vi "Pade_filter_parameters.vi"(7 "Cheby constraints":bool=TRUE, 10 "order cluster":cluster{u32, i32, i32}[][][](array[cluster])=[[[{3, 2, 2}, {3, 2, 1}, {0, 0, 0}, {0, 0, 0}, {0, 0, 0}, {0, 0, 0}, {0, 0, 0}], [{3, 3, 3}, {3, 3, 2}, {3, 3, 1}, {0, 0, 0}, {0, 0, 0}, {0, 0, 0}, {0, 0, 0}], [{3, 4, 4}, {3, 4, 3}, {3, 4, 2}, {3, 4, 1}, {0, 0, 0}, {0, 0, 0}, {0, 0, 0}], [{3, 5, 5}, {3, 5, 4}, {3, 5, 3}, {3, 5, 2}, {3, 5, 1}, {0, 0, 0}, {0, 0, 0}], [{3, 6, 6}, {3, 6, 5}, {3, 6, 4}, {3, 6, 3}, {3, 6, 2}, {3, 6, 1}, {0, 0, 0}], [{3, 7, 7}, {3, 7, 6}, {3, 7, 5}, {3, 7, 4}, {3, 7, 3}, {3, 7, 2}, {3, 7, 1}]], [[{4, 2, 2}, {4, 2, 1}, {0, 0, 0}, {0, 0, 0}, {0, 0, 0}, {0, 0, 0}, {0, 0, 0}], [{4, 3, 3}, {4, 3, 2}, {4, 3, 1}, {0, 0, 0}, {0, 0, 0}, {0, 0, 0}, {0, 0, 0}], [{4, 4, 4}, {4, 4, 3}, {4, 4, 2}, {4, 4, 1}, {0, 0, 0}, {0, 0, 0}, {0, 0, 0}], [{4, 5, 5}, {4, 5, 4}, {4, 5, 3}, {4, 5, 2}, {4, 5, 1}, {0, 0, 0}, {0, 0, 0}], [{4, 6, 6}, {4, 6, 5}, {4, 6, 4}, {4, 6, 3}, {4, 6, 2}, {4, 6, 1}, {0, 0, 0}], [{4, 7, 7}, {4, 7, 6}, {4, 7, 5}, {4, 7, 4}, {4, 7, 3}, {4, 7, 2}, {4, 7, 1}]], [[{5, 2, 2}, {5, 2, 1}, {0, 0, 0}, {0, 0, 0}, {0, 0, 0}, {0, 0, 0}, {0, 0, 0}], [{5, 3, 3}, {5, 3, 2}, {5, 3, 1}, {0, 0, 0}, {0, 0, 0}, {0, 0, 0}, {0, 0, 0}], [{5, 4, 4}, {5, 4, 3}, {5, 4, 2}, {5, 4, 1}, {0, 0, 0}, {0, 0, 0}, {0, 0, 0}], [{5, 5, 5}, {5, 5, 4}, {5, 5, 3}, {5, 5, 2}, {5, 5, 1}, {0, 0, 0}, {0, 0, 0}], [{5, 6, 6}, {5, 6, 5}, {5, 6, 4}, {5, 6, 3}, {5, 6, 2}, {5, 6, 1}, {0, 0, 0}], [{5, 7, 7}, {5, 7, 6}, {5, 7, 5}, {5, 7, 4}, {5, 7, 3}, {5, 7, 2}, {5, 7, 1}]], [[{6, 2, 2}, {6, 2, 1}, {0, 0, 0}, {0, 0, 0}, {0, 0, 0}, {0, 0, 0}, {0, 0, 0}], [{6, 3, 3}, {6, 3, 2}, {6, 3, 1}, {0, 0, 0}, {0, 0, 0}, {0, 0, 0}, {0, 0, 0}], [{6, 4, 4}, {6, 4, 3}, {6, 4, 2}, {6, 4, 1}, {0, 0, 0}, {0, 0, 0}, {0, 0, 0}], [{6, 5, 5}, {6, 5, 4}, {6, 5, 3}, {6, 5, 2}, {6, 5, 1}, {0, 0, 0}, {0, 0, 0}], [{6, 6, 6}, {6, 6, 5}, {6, 6, 4}, {6, 6, 3}, {6, 6, 2}, {6, 6, 1}, {0, 0, 0}], [{6, 7, 7}, {6, 7, 6}, {6, 7, 5}, {6, 7, 4}, {6, 7, 3}, {6, 7, 2}, {6, 7, 1}]], [[{7, 2, 2}, {7, 2, 1}, {0, 0, 0}, {0, 0, 0}, {0, 0, 0}, {0, 0, 0}, {0, 0, 0}], [{7, 3, 3}, {7, 3, 2}, {7, 3, 1}, {0, 0, 0}, {0, 0, 0}, {0, 0, 0}, {0, 0, 0}], [{7, 4, 4}, {7, 4, 3}, {7, 4, 2}, {7, 4, 1}, {0, 0, 0}, {0, 0, 0}, {0, 0, 0}], [{7, 5, 5}, {7, 5, 4}, {7, 5, 3}, {7, 5, 2}, {7, 5, 1}, {0, 0, 0}, {0, 0, 0}], [{7, 6, 6}, {7, 6, 5}, {7, 6, 4}, {7, 6, 3}, {7, 6, 2}, {7, 6, 1}, {0, 0, 0}], [{7, 7, 7}, {7, 7, 6}, {7, 7, 5}, {7, 7, 4}, {7, 7, 3}, {7, 7, 2}, {7, 7, 1}]], [[{8, 2, 2}, {8, 2, 1}, {0, 0, 0}, {0, 0, 0}, {0, 0, 0}, {0, 0, 0}, {0, 0, 0}], [{8, 3, 3}, {8, 3, 2}, {8, 3, 1}, {0, 0, 0}, {0, 0, 0}, {0, 0, 0}, {0, 0, 0}], [{8, 4, 4}, {8, 4, 3}, {8, 4, 2}, {8, 4, 1}, {0, 0, 0}, {0, 0, 0}, {0, 0, 0}], [{8, 5, 5}, {8, 5, 4}, {8, 5, 3}, {8, 5, 2}, {8, 5, 1}, {0, 0, 0}, {0, 0, 0}], [{8, 6, 6}, {8, 6, 5}, {8, 6, 4}, {8, 6, 3}, {8, 6, 2}, {8, 6, 1}, {0, 0, 0}], [{8, 7, 7}, {8, 7, 6}, {8, 7, 5}, {8, 7, 4}, {8, 7, 3}, {8, 7, 2}, {8, 7, 1}]], [[{9, 2, 2}, {9, 2, 1}, {0, 0, 0}, {0, 0, 0}, {0, 0, 0}, {0, 0, 0}, {0, 0, 0}], [{9, 3, 3}, {9, 3, 2}, {9, 3, 1}, {0, 0, 0}, {0, 0, 0}, {0, 0, 0}, {0, 0, 0}], [{9, 4, 4}, {9, 4, 3}, {9, 4, 2}, {9, 4, 1}, {0, 0, 0}, {0, 0, 0}, {0, 0, 0}], [{9, 5, 5}, {9, 5, 4}, {9, 5, 3}, {9, 5, 2}, {9, 5, 1}, {0, 0, 0}, {0, 0, 0}], [{9, 6, 6}, {9, 6, 5}, {9, 6, 4}, {9, 6, 3}, {9, 6, 2}, {9, 6, 1}, {0, 0, 0}], [{9, 7, 7}, {9, 7, 6}, {9, 7, 5}, {9, 7, 4}, {9, 7, 3}, {9, 7, 2}, {9, 7, 1}]], [[{10, 2, 2}, {10, 2, 1}, {0, 0, 0}, {0, 0, 0}, {0, 0, 0}, {0, 0, 0}, {0, 0, 0}], [{10, 3, 3}, {10, 3, 2}, {10, 3, 1}, {0, 0, 0}, {0, 0, 0}, {0, 0, 0}, {0, 0, 0}], [{10, 4, 4}, {10, 4, 3}, {10, 4, 2}, {10, 4, 1}, {0, 0, 0}, {0, 0, 0}, {0, 0, 0}], [{10, 5, 5}, {10, 5, 4}, {10, 5, 3}, {10, 5, 2}, {10, 5, 1}, {0, 0, 0}, {0, 0, 0}], [{10, 6, 6}, {10, 6, 5}, {10, 6, 4}, {10, 6, 3}, {10, 6, 2}, {10, 6, 1}, {0, 0, 0}], [{10, 7, 7}, {10, 7, 6}, {10, 7, 5}, {10, 7, 4}, {10, 7, 3}, {10, 7, 2}, {10, 7, 1}]], [[{11, 2, 2}, {11, 2, 1}, {0, 0, 0}, {0, 0, 0}, {0, 0, 0}, {0, 0, 0}, {0, 0, 0}], [{11, 3, 3}, {11, 3, 2}, {11, 3, 1}, {0, 0, 0}, {0, 0, 0}, {0, 0, 0}, {0, 0, 0}], [{11, 4, 4}, {11, 4, 3}, {11, 4, 2}, {11, 4, 1}, {0, 0, 0}, {0, 0, 0}, {0, 0, 0}], [{11, 5, 5}, {11, 5, 4}, {11, 5, 3}, {11, 5, 2}, {11, 5, 1}, {0, 0, 0}, {0, 0, 0}], [{11, 6, 6}, {11, 6, 5}, {11, 6, 4}, {11, 6, 3}, {11, 6, 2}, {11, 6, 1}, {0, 0, 0}], [{11, 7, 7}, {11, 7, 6}, {11, 7, 5}, {11, 7, 4}, {11, 7, 3}, {11, 7, 2}, {11, 7, 1}]]], 11 "Array":dbl[][][](array[numeric])=[[[0.002353454560863419, 0.007689391633254067, 99.0, 99.0, 99.0, 99.0, 99.0], [0.0023534545608634183, 0.0023534545608634183, nan, 99.0, 99.0, 99.0, 99.0], [0.002353454560863419, 0.0023534545608634187, 0.0023534545608634165, nan, 99.0, 99.0, 99.0], [0.0023534545608634187, 0.0023534545608634126, 0.0023534545608634187, nan, nan, 99.0, 99.0], [0.002353454560863415, 0.0023534545608634196, 0.0023534545608634187, 0.0023534545608634187, nan, nan, 99.0], [0.0023534545608634196, 0.0023534545608634187, 0.002353454560863419, 0.0023534545608634217, nan, nan, nan]], [[0.00371393896279979, 0.002290524417185622, 99.0, 99.0, 99.0, 99.0, 99.0], [0.0017925839925326166, 0.002655859928068269, nan, 99.0, 99.0, 99.0, 99.0], [0.0017925839925326172, 0.0017925839925326174, 0.0023176227448640247, nan, 99.0, 99.0, 99.0], [0.0017925839925326174, 0.001792583992532618, 0.0017925839925326166, nan, nan, 99.0, 99.0], [0.0017925839925326177, 0.001792583992532617, 0.0017925839925326168, 0.001792583992532617, nan, nan, 99.0], [0.001792583992532617, 0.0017925839925326168, 0.001792583992532617, 0.0017925839925326203, nan, nan, nan]], [[0.006335862370584556, 4.598350317328608, 99.0, 99.0, 99.0, 99.0, 99.0], [0.004085329918918175, 0.006093286554374381, nan, 99.0, 99.0, 99.0, 99.0], [0.0009130542045032324, 1.1358755116875932, 0.006420203154987485, nan, 99.0, 99.0, 99.0], [0.0009130542045032329, 0.0009130542045032349, 0.001335233103777126, nan, nan, 99.0, 99.0], [0.0009130542045032358, 0.0009130542045032318, 0.0009130542045032328, 0.0014881550617160033, nan, nan, 99.0], [0.0009130542045032318, 0.0009130542045032327, 0.0009130542045032316, 0.0009130542045032325, nan, nan, nan]], [[0.005445709835049192, 3.1805644316751045, 99.0, 99.0, 99.0, 99.0, 99.0], [0.007126719886814989, 0.0077277729414607635, nan, 99.0, 99.0, 99.0, 99.0], [0.0050356545643726715, 0.207214492171318, 0.004878014522941635, nan, 99.0, 99.0, 99.0], [0.0006116453626043867, 0.011523702553404421, 0.002782034706759067, nan, nan, 99.0, 99.0], [0.0006116453626043876, 0.0006116453626043851, 0.0018983210716558261, 0.0013504416986585758, nan, nan, 99.0], [0.0006116453626043851, 0.0006116453626043848, 0.0006116453626043852, 0.042137479943127505, nan, nan, nan]], [[0.0036052378399916863, 0.03348457198286975, 99.0, 99.0, 99.0, 99.0, 99.0], [0.006552878510569864, 0.008226196723185418, nan, 99.0, 99.0, 99.0, 99.0], [0.006588705257043203, 0.006590513691825371, 0.006176591916597983, nan, 99.0, 99.0, 99.0], [0.0032285973888167047, 0.006554231155519152, 0.010964671813698309, nan, nan, 99.0, 99.0], [0.00045863692336361913, 0.005674419947933448, 0.004062500092018482, 0.003087609801193326, nan, nan, 99.0], [0.0004586369233636209, 0.0004586369233636214, 0.0014784335573549642, 0.0026992398485220204, nan, nan, nan]], [[0.004366303750002497, 0.03706707255474952, 99.0, 99.0, 99.0, 99.0, 99.0], [0.002820062475467122, 0.006561477198178083, nan, 99.0, 99.0, 99.0, 99.0], [0.0046981751026274055, 0.006572929421810439, 0.006572905249549529, nan, 99.0, 99.0, 99.0], [0.006897571176760764, 0.053891672701654035, 0.0065614821654988035, nan, nan, 99.0, 99.0], [0.005328270847333867, 0.020376055012549743, 0.0032997310552627117, 0.08822873403893636, nan, nan, 99.0], [0.0003856734622259503, 1.1066269871712326, 0.0035594095050575777, 0.003637060326888666, nan, nan, nan]], [[0.006059291579447172, 1.680187711493279, 99.0, 99.0, 99.0, 99.0, 99.0], [0.005199838175639393, 0.006592168144080282, nan, 99.0, 99.0, 99.0, 99.0], [0.006113912994155667, 0.011716550829946054, 0.010601186501658037, nan, 99.0, 99.0, 99.0], [0.008748300547543142, 0.014757438954492452, 0.002118890522388517, nan, nan, 99.0, 99.0], [0.01076329870877188, 0.022398438235242728, 0.0020245436197548297, 0.0019095225881288643, nan, nan, 99.0], [0.008649122742919929, 0.01115622666481453, 0.003062796349276221, 0.013155279374776592, nan, nan, nan]], [[0.0025815412910655837, 0.009241241231513755, 99.0, 99.0, 99.0, 99.0, 99.0], [0.008249512431695302, 0.022432753781857113, nan, 99.0, 99.0, 99.0, 99.0], [0.010810117988469183, 0.7061514210645411, 1.0546374871859439, nan, 99.0, 99.0, 99.0], [0.011597246304021924, 0.022309928750349328, 0.02661676478748557, nan, nan, 99.0, 99.0], [0.009263594144453215, 0.020755452243573898, 0.004844928434400263, 0.026953885057255902, nan, nan, 99.0], [0.00781382060949307, 0.24691358561267165, 0.0036580354189426887, 0.00734741345514906, nan, nan, nan]], [[0.004842715718191497, 2.2110947302495303, 99.0, 99.0, 99.0, 99.0, 99.0], [0.0038566413732330257, 0.00408648546930453, nan, 99.0, 99.0, 99.0, 99.0], [0.009569457748718148, 0.005011628382040588, 0.014308799751274918, nan, 99.0, 99.0, 99.0], [0.009504820050901041, 0.009525366540292513, 0.002785528891405663, nan, nan, 99.0, 99.0], [0.030452371081413385, 0.00957637575444143, 0.002612361282403047, 0.001709862367584203, nan, nan, 99.0], [0.030529415641798494, 0.030576778064152172, 0.0016767947139024687, 0.0017328512772866007, nan, nan, nan]]]) -> (3 "Cluster":cluster{u32, i32, i32}={11, 7, 5})   [LabVIEW 2025]
panel:
  out "size(s)":i32[](array[numeric])
  # "Find meaningul Pade parameters"
  # "p=m+n\nm>=n\n\nIf P > Cheby order, the best Pade fitting is same with the result of Cheby-only fitting."
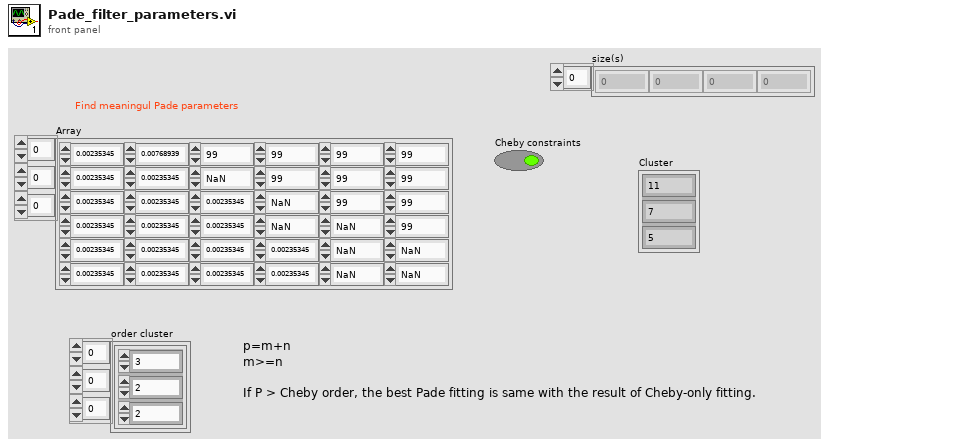
[diagram p1: front panel]
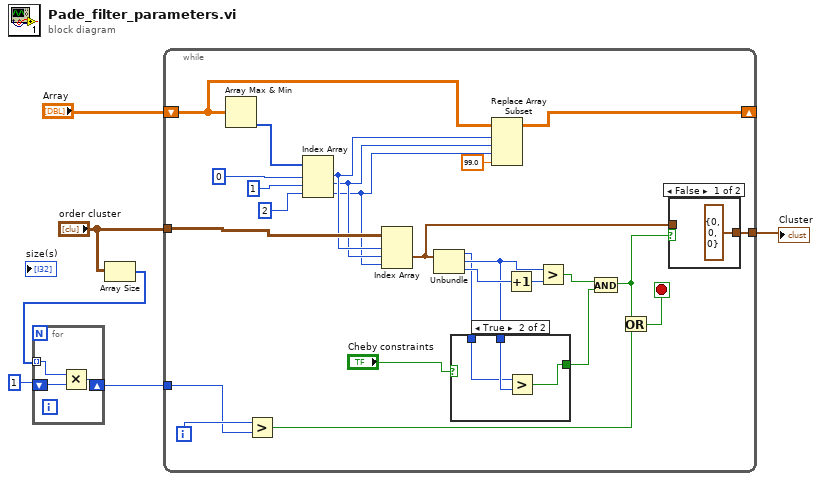
[diagram p0: block diagram]
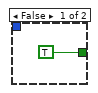
[diagram p3: hidden frame]
diagram:
  n1 = Array Size(array="order cluster") -> (size(s)=w3:i32[])
  n2 = for {
    tunnel: w3 -> [w9] mode=indexing
    shift-right: [w7] -> w1
    shift-left: 1 -> [w8]
    n3 = Multiply(x=w9, y=w8) -> (x*y=w7:i32)
  }
  n4 = while {
    shift-right: [w28] -> _
    shift-left: "Array" -> [w29]
    tunnel: "order cluster" -> [w27]
    tunnel: [w11] -> w5
    tunnel: w1 -> [w15]
    i -> [w16]
    stop <- w14 stop-if-true
    n5 = Array Max & Min(array=w29) -> (min index (indices)=w34:i32[])  [unwired: 3 out]
    n6 = Greater?(x=w16, y=w15) -> (0:w13:bool)
    n7 = Index Array(array=w34, index #1=0 ("index"), index #2=1 ("index"), index #3=2 ("index")) -> (element #1=w26:i32, element #2=w25:i32, element #3=w24:i32)
    n8 = Index Array(array=w27, index (dim 0)=w26, index (dim 1)=w25, index (dim 2)=w24) -> (element=w10:cluster{u32, i32, i32})
    n9 = Unbundle(w10) -> (w17:u32, w18:i32, w23:i32)
    n10 = case shown="True" "Cheby constraints" {
      tunnel: [TRUE ("y") w38] -> w19
      tunnel: w18 -> [_ w40]
      tunnel: w17 -> [_ w39]
      frame False {
      }
      frame True {
        n11 = Greater?(x=w39, y=w40) -> (0:w38:bool)
      }
    }
    n12 = Replace Array Subset(array=w29, new element=99.0 ("new element/subarray"), index (dim 0)=w26, index (dim 1)=w25, index (dim 2)=w24) -> (w28:dbl[][][])
    n13 = Increment(x=w23) -> (x+1=w22:i32)
    n14 = Greater?(x=w18, y=w22) -> (0:w21:bool)
    n15 = And(x=w21, y=w19) -> (x .and. y?=w12:bool)
    n16 = Or(x=w12, y=w13) -> (x .or. y?=w14:bool)
    n17 = case shown="False" w12 {
      tunnel: [cluster{u32, i32, i32} {0, 0, 0} w36] -> w11
      tunnel: w10 -> [_ w36]
      frame False {
      }
      frame True {
      }
    }
  }
  "Cluster" <- w5
